vi "IMMU - Initialise.vi"(8 "error in (no error)":errorcluster) -> (0 "error out":errorcluster, 3 "I2C Ref Out":T1={"myRIO Reference"={"myRIO Model"=enum."Unknown", "myRIO Hardware Reference"={"Generic FPGA Reference"=refnum, "Allow multiple opens"=FALSE}}, "I2C Channels Enum"=enum."Not Connected", "I2C Configuration"={"I2C Transfer Rate"=enum."Fast mode (400 kbps)"}})   [LabVIEW 2021]
uses:
  <vilib>/myRIO/Instrument Drivers/Onboard IO/I2C/typedefs/I2C Reference.ctl
  <vilib>/myRIO/Common/Instrument Driver Framework/Utilities/typedefs/myRIO Generic Hardware Reference.ctl
  <vilib>/myRIO/Common/Instrument Driver Framework/Utilities/typedefs/Hardware Version Enum.ctl
  <vilib>/myRIO/Common/Instrument Driver Framework/Utilities/typedefs/myRIO v1.0 Reference.ctl
  <vilib>/myRIO/Common/Instrument Driver Framework/Utilities/typedefs/Generic FPGA Reference.ctl
  <vilib>/myRIO/Common/Instrument Driver Framework/myRIO v1.0/I2C/typedefs/I2C Channels Enum.ctl
  <vilib>/myRIO/Instrument Drivers/Onboard IO/I2C/typedefs/I2C Configuration.ctl
  <vilib>/myRIO/Instrument Drivers/Onboard IO/I2C/typedefs/I2C Transfer Rate.ctl
  <vilib>/myRIO/Instrument Drivers/Onboard IO/I2C/typedefs/I2C User Configuration.ctl
  <vilib>/Utility/error.llb/Error Cluster From Error Code.vi
  <vilib>/myRIO/Common/Instrument Driver Framework/myRIO v1.0/I2C/vis/myRIO v1.0 Configure I2C.vi
  <vilib>/myRIO/Common/Instrument Driver Framework/myRIO v1.0/I2C/vis/myRIO v1.0 Write I2C.vi
  <vilib>/myRIO/Instrument Drivers/Onboard IO/I2C/I2C.lvlib
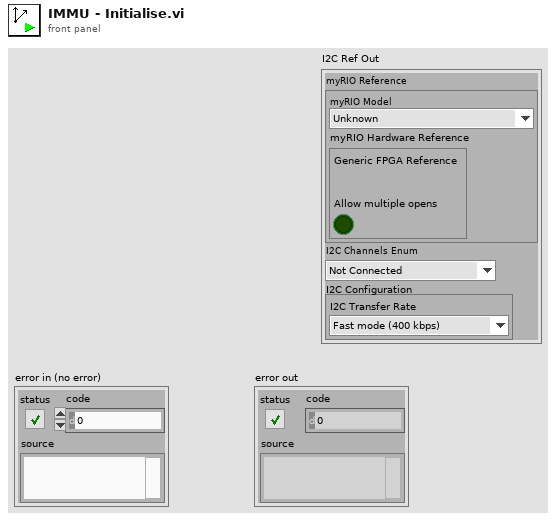
[diagram p1: front panel]
types:
  T1 = typedef "I2C.lvlib/I2C Reference.ctl" = cluster{"myRIO Reference":T2, "I2C Channels Enum":T6, "I2C Configuration":T7}
  T2 = typedef "myRIO Generic Hardware Reference.ctl" = cluster{"myRIO Model":T3, "myRIO Hardware Reference":T4}
  T3 = typedef "Hardware Version Enum.ctl" = enum16{"Unknown", "myRIO-1900", "myRIO-1950", "roboRIO", "NI ELVIS RIO CM", "ELVIS III"}
  T4 = typedef "myRIO v1.0 Reference.ctl" = cluster{"Generic FPGA Reference":T5, "Allow multiple opens":bool}
  T5 = typedef "Generic FPGA Reference.ctl" = refnum<k20>
  T6 = typedef "I2C Channels Enum.ctl" = enum16{"Not Connected", "A/I2C", "B/I2C", "I2C/I2C"}
  T7 = typedef "I2C.lvlib/I2C Configuration.ctl" = cluster{"I2C Transfer Rate":T8}
  T8 = typedef "I2C.lvlib/I2C Transfer Rate.ctl" = enum16{"Standard mode (100 kbps)", "Fast mode (400 kbps)"}
  T9 = typedef "I2C.lvlib/I2C User Configuration.ctl" = cluster{"I2C Transfer Rate":T8}
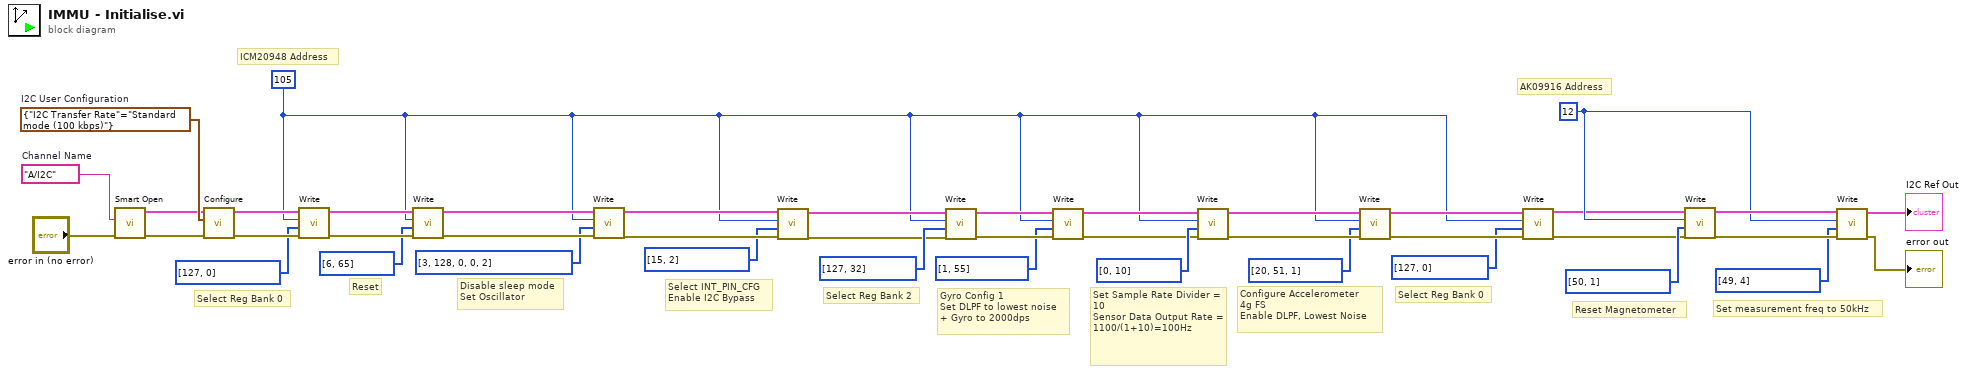
[diagram p0: block diagram]
diagram:
  w9 = u8 12 ("Slave Address (7-bit)")
  w6 = u8 105 ("Slave Address (7-bit)")
  w41 = T9 {"I2C Transfer Rate"=enum."Standard mode (100 kbps)"}  # I2C User Configuration
  w42 = tag "A/I2C"  # Channel Name
  # "Select Reg Bank 0"
  # "AK09916 Address"
  # "Select INT_PIN_CFG\nEnable I2C Bypass"
  # "Configure Accelerometer\n4g FS\nEnable DLPF, Lowest Noise"
  # "Set Sample Rate Divider = 10\nSensor Data Output Rate = 1100/(1+10)=100Hz"
  # "Gyro Config 1\nSet DLPF to lowest noise\n+ Gyro to 2000dps"
  # "ICM20948 Address"
  # "Disable sleep mode\nSet Oscillator"
  # "Reset"
  # "Select Reg Bank 0"
  # "Set measurement freq to 50kHz"
  # "Reset Magnetometer"
  # "Select Reg Bank 2"
  n1 = call <vilib>:"Smart Open.vi"("error in (no error)"="error in (no error)", "Channel Name"=w42) -> ("error out"=w39:errorcluster, "I2C Ref Out"=w40:T1)  [unwired: 8 in]
  n2 = call <vilib>:"Configure.vi"("error in (no error)"=w39, "I2C User Configuration"=w41, "I2C Ref In"=w40) -> ("error out"=w37:errorcluster, "I2C Ref Out"=w38:T1)  [unwired: 7 in]
  n3 = call <vilib>:"Write.vi"("error in (no error)"=w37, "Bytes to Write"=u8[] [127, 0], "Slave Address (7-bit)"=w6, "I2C Ref In"=w38) -> ("error out"=w33:errorcluster, "I2C Ref Out"=w34:T1)  [unwired: 6 in]
  n4 = call <vilib>:"Write.vi"("error in (no error)"=w33, "Bytes to Write"=u8[] [6, 65], "Slave Address (7-bit)"=w6, "I2C Ref In"=w34) -> ("error out"=w30:errorcluster, "I2C Ref Out"=w31:T1)  [unwired: 6 in]
  n5 = call <vilib>:"Write.vi"("error in (no error)"=w30, "Bytes to Write"=u8[] [3, 128, 0, 0, 2], "Slave Address (7-bit)"=w6, "I2C Ref In"=w31) -> ("error out"=w17:errorcluster, "I2C Ref Out"=w18:T1)  [unwired: 6 in]
  n6 = call <vilib>:"Write.vi"("error in (no error)"=w17, "Bytes to Write"=u8[] [15, 2], "Slave Address (7-bit)"=w6, "I2C Ref In"=w18) -> ("error out"=w16:errorcluster, "I2C Ref Out"=w15:T1)  [unwired: 6 in]
  n7 = call <vilib>:"Write.vi"("error in (no error)"=w16, "Bytes to Write"=u8[] [127, 32], "Slave Address (7-bit)"=w6, "I2C Ref In"=w15) -> ("error out"=w26:errorcluster, "I2C Ref Out"=w27:T1)  [unwired: 6 in]
  n8 = call <vilib>:"Write.vi"("error in (no error)"=w26, "Bytes to Write"=u8[] [1, 55], "Slave Address (7-bit)"=w6, "I2C Ref In"=w27) -> ("error out"=w23:errorcluster, "I2C Ref Out"=w22:T1)  [unwired: 6 in]
  n9 = call <vilib>:"Write.vi"("error in (no error)"=w23, "Bytes to Write"=u8[] [0, 10], "Slave Address (7-bit)"=w6, "I2C Ref In"=w22) -> ("error out"=w20:errorcluster, "I2C Ref Out"=w21:T1)  [unwired: 6 in]
  n10 = call <vilib>:"Write.vi"("error in (no error)"=w20, "Bytes to Write"=u8[] [20, 51, 1], "Slave Address (7-bit)"=w6, "I2C Ref In"=w21) -> ("error out"=w7:errorcluster, "I2C Ref Out"=w8:T1)  [unwired: 6 in]
  n11 = call <vilib>:"Write.vi"("error in (no error)"=w7, "Bytes to Write"=u8[] [127, 0], "Slave Address (7-bit)"=w6, "I2C Ref In"=w8) -> ("error out"=w3:errorcluster, "I2C Ref Out"=w4:T1)  [unwired: 6 in]
  n12 = call <vilib>:"Write.vi"("error in (no error)"=w3, "Bytes to Write"=u8[] [50, 1], "Slave Address (7-bit)"=w9, "I2C Ref In"=w4) -> ("error out"=w11:errorcluster, "I2C Ref Out"=w12:T1)  [unwired: 6 in]
  n13 = call <vilib>:"Write.vi"("error in (no error)"=w11, "Bytes to Write"=u8[] [49, 4], "Slave Address (7-bit)"=w9, "I2C Ref In"=w12) -> ("error out"=→"error out":errorcluster, "I2C Ref Out"=→"I2C Ref Out":T1)  [unwired: 6 in]
